vi "Read NISTWfrmModuleID.vi"(8 "error in (no error)":errorcluster, 11 "NISTBus in":refnum<class "NISTBus.lvclass">) -> (0 "error out":errorcluster, 2 "NISTWfrmModuleID":i32, 3 "NISTBus out":refnum<class "NISTBus.lvclass">)   [LabVIEW 2014, in "Bus.lvlib" / "NISTBus.lvclass"]
uses:
  Test/Bus/NISTBus.lvclass
  Test/Bus/NISTBus.lvclass/NISTBus.ctl
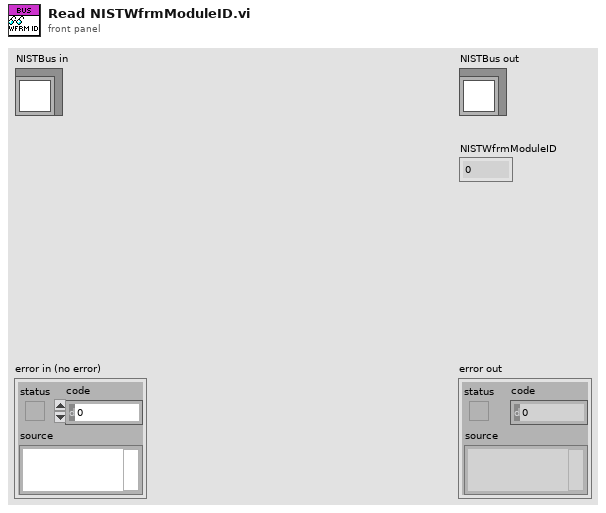
[diagram p1: front panel]
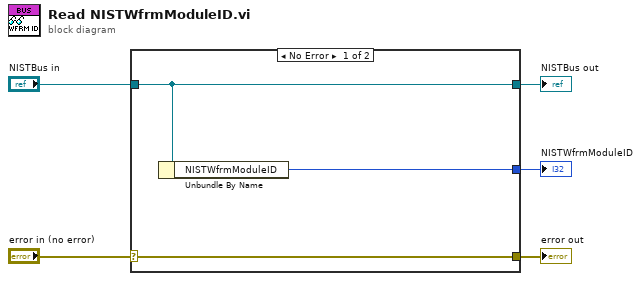
[diagram p0: block diagram]
diagram:
  n1 = case shown="No Error" "error in (no error)" {
    selector: "error in (no error)" -> [w8 w9]
    tunnel: [w8 w9] -> w4
    tunnel: [w7 w10] -> w2
    tunnel: "NISTBus in" -> [w7 w10]
    tunnel: [w6 _] -> w1
    frame No Error {
      n2 = Unbundle By Name(w7) -> ("NISTWfrmModuleID"=w6:i32)
    }
    frame Error {
    }
  }
  "error out" <- w4
  "NISTBus out" <- w2
  "NISTWfrmModuleID" <- w1
